vi "Example Threshold.vi"() -> ()   [LabVIEW 2013]
uses:
  C:/tf/play/labview/Tinkerforge.dll
  Tinkerforge.dll
panel:
  in  "stop":bool
  out "callback counter":i32
  out "last current (mA)":sgl
  in  "uid":string="amb"
  in  "port":i32=4223
  in  "host":string="localhost"
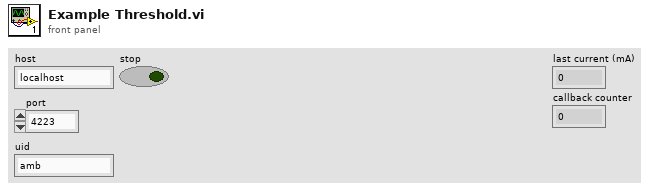
[diagram p1: front panel]
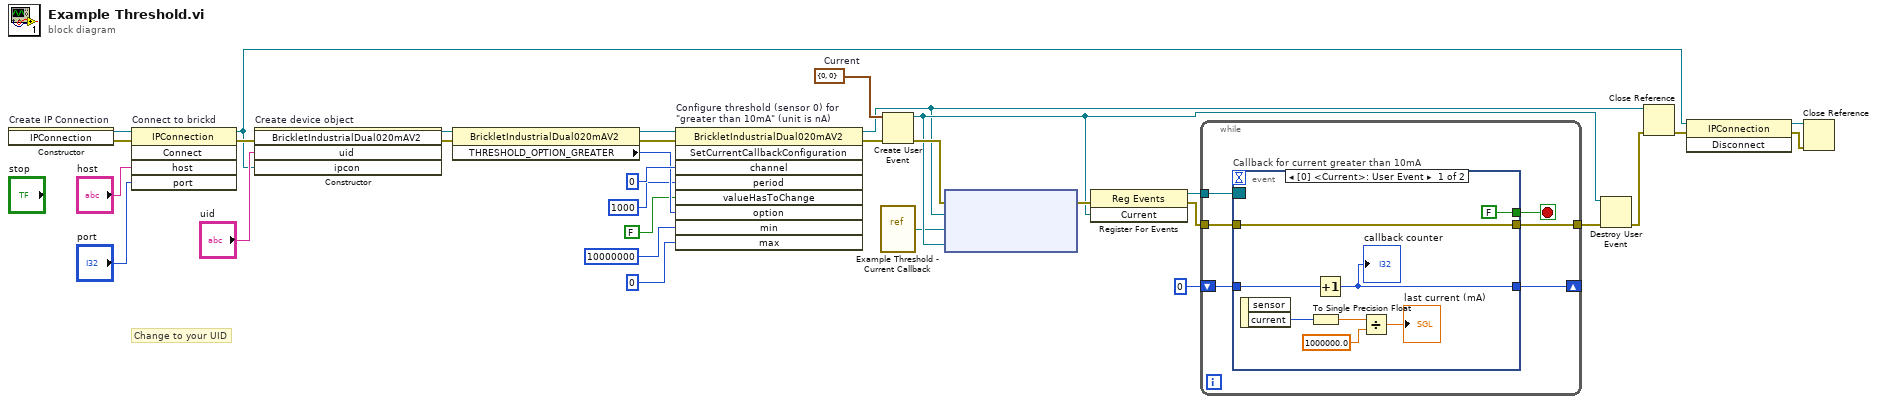
[diagram p0: block diagram]
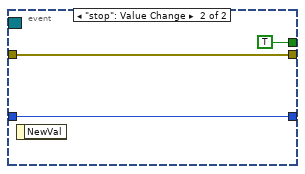
[diagram p2: hidden frame]
diagram:
  w16 = cluster{"sensor":u8, "current":i32} {"sensor"=0, "current"=0}  # Current
  # "Change to your UID"
  n1 = constructor on="Create IP Connection" class="IPConnection"() -> (reference out=w32:refnum<k24>, error out=w10:errorcluster)  [unwired: 3 in, 1 out]
  n2 = invoke on="Connect to brickd" class="IPConnection" method="Connect"(reference=w32, error in=w10, "host"="host", "port"="port") -> (reference out=w25:refnum<k24>, error out=w28:errorcluster)  [unwired: 1 in, 3 out]
  n3 = constructor on="Create device object" class="BrickletIndustrialDual020mAV2"(error in=w28, "uid"="uid", "ipcon"=w25) -> (reference out=w7:refnum<k24>, error out=w8:errorcluster)  [unwired: 2 in, 3 out]
  n4 = property class="BrickletIndustrialDual020mAV2"(reference=w7, error in=w8) -> (reference out=w12:refnum<k24>, error out=w13:errorcluster, "THRESHOLD_OPTION_GREATER"=w4:u16)
  n5 = invoke on="Configure threshold (sensor 0) for\n\"greater than 10mA\" (unit is nA)" class="BrickletIndustrialDual020mAV2" method="SetCurrentCallbackConfiguration"(reference=w12, error in=w13, "channel"=u8 0 ("sensor"), "period"=i64 1000, "valueHasToChange"=FALSE, "option"=w4, "min"=10000000, "max"=0) -> (reference out=w15:refnum<k24>, error out=w14:errorcluster)  [unwired: 1 in, 7 out]
  n6 = vi-ref "Example Threshold - Current Callback.vi"() -> ("vi reference"=w2:refnum<vi>)
  n7 = Create User Event(user event datatype=w16, error in=w14) -> (user event=w18:refnum<user-event>, error out=w23:errorcluster)
  n8 = node ("Register Event Callback")(w23, w15, w2, w18) -> (w22:errorcluster)  [unwired: 1 in, 1 out]
  n9 = register-events(error in=w22, w18) -> (reference out=w21:refnum<event-registration>, error out=w19:errorcluster)  [unwired: 1 in]
  n10 = while {
    tunnel: w21 -> [w38]
    tunnel: [w37] -> w20
    tunnel: w19 -> [w36]
    shift-right: [w34] -> _
    shift-left: 0 -> [w35]
    stop <- w33 stop-if-true
    n11 = event "Callback for current greater than 10mA" shown="[0] <Current>: User Event" {
      selector: w38 -> [_ _]
      dyn-events: _ -> [_ _]
      timeout: _ -> [_ _]
      tunnel: [w43 w48] -> w37
      tunnel: w36 -> [w43 w48]
      tunnel: w35 -> [w41 w47]
      tunnel: [w40 w47] -> w34
      tunnel: [FALSE TRUE] -> w33
      event User Event {
        n12 = event-data() -> ("current"=w44:i32)  [unwired: 1 in, 1 out]
        n13 = To Single Precision Float(number=w44) -> (single precision float=w45:sgl)
        n14 = Increment(x=w41) -> (x+1=w40:i32)
        "callback counter" <- w40
        n15 = Divide(x=w45, y=sgl 1000000.0) -> (x/y=→"last current (mA)":sgl)
      }
      event "stop": Value Change {
        n16 = event-data() -> ()  [unwired: 1 in, 1 out]
      }
    }
  }
  n17 = Destroy User Event(user event=w18, error in=w20) -> (error out=w17:errorcluster)
  n18 = Close Reference(reference=w15, error in (no error)=w17) -> (error out=w27:errorcluster)
  n19 = invoke class="IPConnection" method="Disconnect"(reference=w25, error in=w27) -> (reference out=w24:refnum<k24>, error out=w26:errorcluster)  [unwired: 1 in, 1 out]
  n20 = Close Reference(reference=w24, error in (no error)=w26) -> ()  [unwired: 1 out]
